vi "Repulsive Force.vi"(9 "Target":dbl[](array[numeric]), 10 "Robot Position":dbl[](array[numeric])) -> (2 "out":dbl[](array[numeric]))   [LabVIEW 2016]
panel:
  in  "gain":dbl=3.0 format="%#_13g"
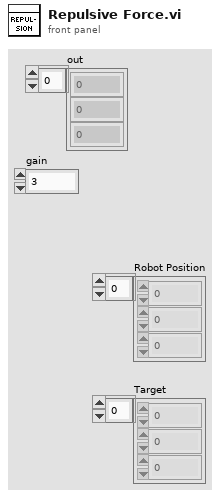
[diagram p1: front panel]
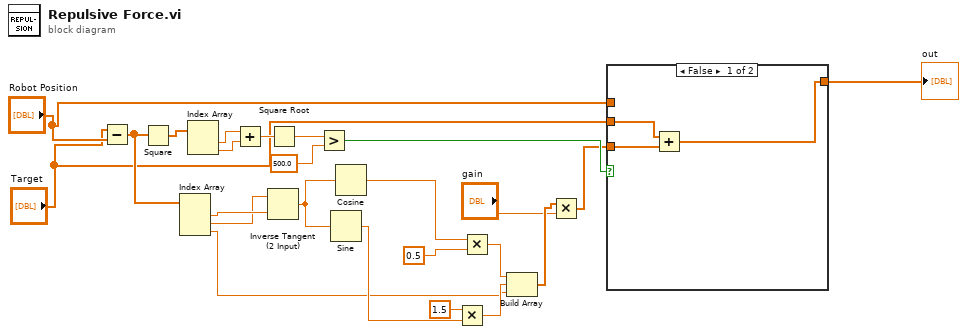
[diagram p0: block diagram]
diagram:
  n1 = Subtract(x="Target", y="Robot Position") -> (x-y=w20:dbl[])
  n2 = Square(x=w20) -> (x^2=w24:dbl[])
  n3 = Index Array(array=w20) -> (element #1=w19:dbl, element #2=w18:dbl, element #3=w6:dbl)  [unwired: 3 in]
  n4 = Index Array(array=w24) -> (element #1=w23:dbl, element #2=w22:dbl)  [unwired: 2 in]
  n5 = Add(x=w23, y=w22) -> (x+y=w21:dbl)
  n6 = Inverse Tangent (2 Input)(1:w19, 2:w18) -> (0:w11:dbl)
  n7 = Square Root(x=w21) -> (sqrt(x)=w17:dbl)
  n8 = Greater?(x=w17, y=500.0) -> (0:w15:bool)
  n9 = Sine(x=w11) -> (sin(x)=w9:dbl)
  n10 = Cosine(x=w11) -> (cos(x)=w10:dbl)
  n11 = Multiply(x=1.5 ("y"), y=w9) -> (x*y=w7:dbl)
  n12 = Multiply(x=w10, y=0.5) -> (x*y=w8:dbl)
  n13 = Build Array(w8, w7, w6) -> (w3:dbl[])
  n14 = Multiply(x=w3, y="gain") -> (x*y=w2:dbl[])
  n15 = case shown="False" w15 {
    tunnel: "Robot Position" -> [_ w28]
    tunnel: [w26 w28] -> w13
    tunnel: w2 -> [w27 _]
    tunnel: "Target" -> [w25 _]
    frame False {
      n16 = Add(x=w25, y=w27) -> (x+y=w26:dbl[])
    }
    frame True {
    }
  }
  "out" <- w13
